vi "Serial Test Controller.vi"() -> ()   [LabVIEW 2012]
uses:
  Type/_RT Serial Command.ctl
  Type/_RT Command.ctl
  <vilib>/Utility/config.llb/Read Key (String).vi
  <vilib>/Utility/config.llb/NI_LVConfig.lvlib
panel:
  in  "Serial Property":T1[](array[typedef])=[{"Port Type"=0, "baud rate (9600)"=9600, "data bits (8)"=8, "stop bits (1)"=10, "parity (0:none)"=0, "DoRead"=TRUE, "Command"=""}, {"Port Type"=1, "baud rate (9600)"=9600, "data bits (8)"=8, "stop bits (1)"=10, "parity (0:none)"=0, "DoRead"=TRUE, "Command"=""}, {"Port Type"=2, "baud rate (9600)"=9600, "data bits (8)"=8, "stop bits (1)"=10, "parity (0:none)"=0, "DoRead"=TRUE, "Command"=""}] {"stop bits (1)" items=["1 bit"=10, "1.5 bits"=15, "2 bits"=20]; "parity (0:none)" items=["None", "Odd", "Even", "Mark", "Space"]; "data bits (8)" min=5 max=8 step=1; "Port Type" items=["RS485", "RS232-1", "RS232-2"]}
  in  "Tab":T2(tab)
  out "Reply":string
  in  "Command":string
  in  "Serial Port":u16(ring) items=["RS485", "RS232-1", "RS232-2"]
  in  "baud rate":u32=9600
  in  "parity":u16(ring) items=["None", "Odd", "Even", "Mark", "Space"]
  in  "stop bits":u16(ring)=10 items=["1 bit"=10, "1.5 bits"=15, "2 bits"=20]
  in  "data bits":u16=8 min=5 max=8 step=1
  in  "Send":bool
  in  "LC1 - Out1":bool
  in  "LC1 - Out2":bool
  in  "LC2 - Out1":bool
  in  "LC2 - Out2":bool
  out "LC1 - In":bool
  out "LC2 - In":bool
  in  "Update":bool
  in  "Read VAC":bool
  out "VAC Gauge Reading":i32
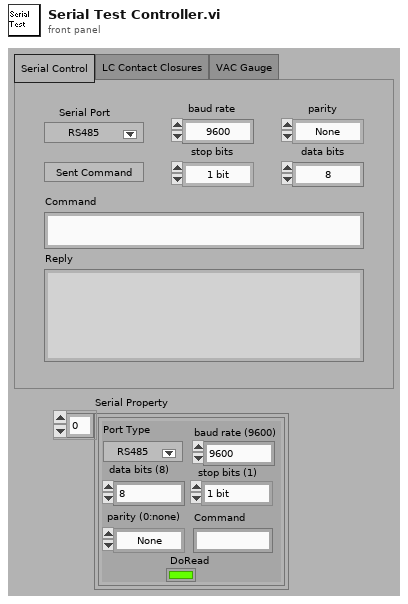
[diagram p1: front panel]
types:
  T1 = typedef "_RT Serial Command.ctl" = cluster{"Port Type":u16, "baud rate (9600)":u32, "data bits (8)":u16, "stop bits (1)":u16, "parity (0:none)":u16, "DoRead":bool, "Command":string}
  T2 = enum32{"Serial Control", "LC Contact Closures", "VAC Gauge"}
  T3 = typedef "_RT Command.ctl" = enum16{"Start", "Stop", "Runtime Update", "Get Data", "Get Info", "Get Status", "Get Param", "Get Config", "Get Table", "Read ADC", "Set Oscillator", "Update Config", "Update Table", "Set All Pol", "Set Pol and DC", "Set Max Mass", "Toggle RP", "Toggle EL", "Set PIC", "Initialize Turbo", "Send Turbo Comm", "Close Turbo", "P1", "P2", "P3", "Send Serial", "Set LC Out", "Get LC In", "Read VAC", "Test Table", "Toggle Power", "Get Startup", "Set Startup", "Get ADC Table", "Set ADC Table", "Get Brief Status", "Get Detail Status", "Auxiliary Update", "Set CC Logics", "Set CC Input Logics", "Ignore Error"}
  T4 = typedef "NI_LVConfig.lvlib/Config Data RefNum.ctl" = refnum<k1>
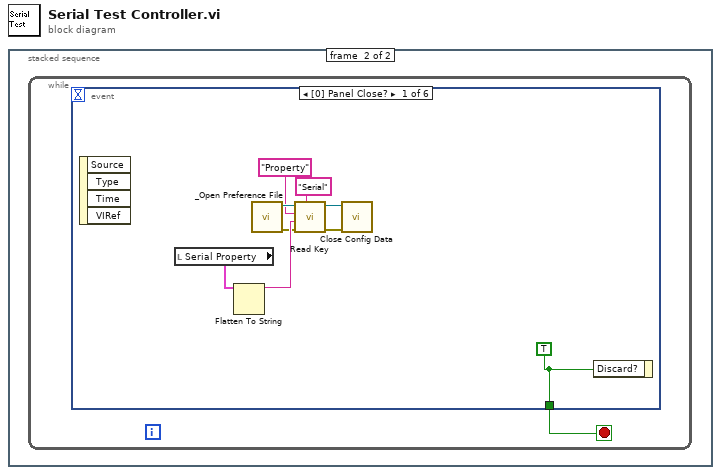
[diagram p0: block diagram]
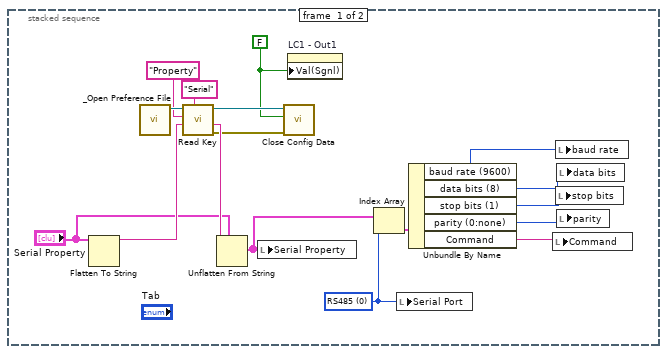
[diagram p2: hidden frame]
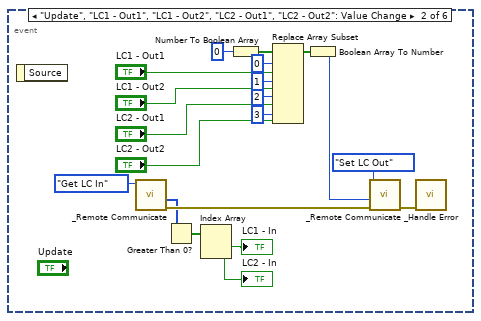
[diagram p3: hidden frame]
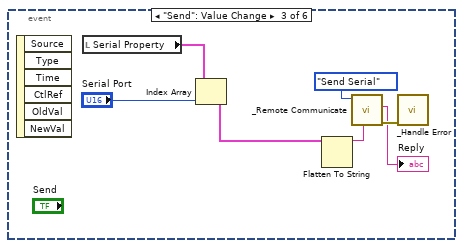
[diagram p4: hidden frame]
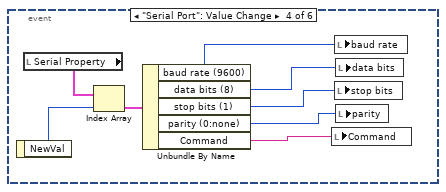
[diagram p5: hidden frame]
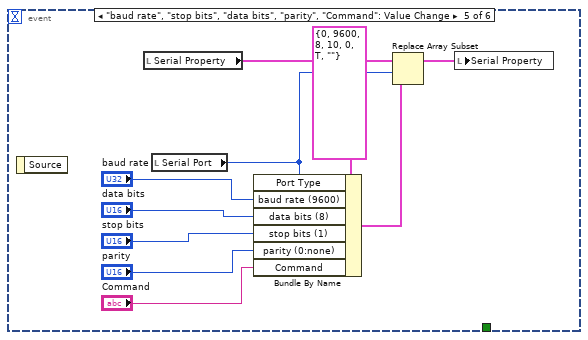
[diagram p6: hidden frame]
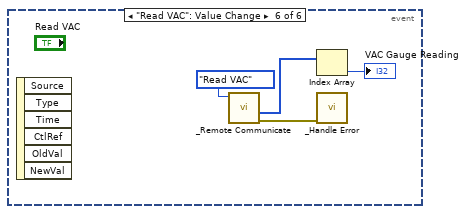
[diagram p7: hidden frame]
diagram:
  n1 = stacked-sequence {
    frame #0 {
      w7 = u16 0 items=["RS485", "RS232-1", "RS232-2"] ("Serial Port")
      w9 = FALSE ("write configuration file? (T)")
      n2 = Flatten To String(anything="Serial Property") -> (data string=w14:string)  [unwired: 1 in, 4 out]
      n3 = call "_Open Preference File.vi"() -> ("refnum"=w17:T4)  [unwired: 1 in, 6 out]
      n4 = call-poly <vilib>:"Read Key.vi"("section"="Serial", "default value"=w14, "key"="Property" ("section"), "refnum"=w17) -> ("error out"=w10:errorcluster, "value"=w13:string, "refnum out"=w11:T4)  [unwired: 2 in, 3 out]
      n5 = Unflatten From String(type="Serial Property", binary string=w13) -> (value=w8:T1[])  [unwired: 1 in, 4 out]
      n6 = local write "Serial Property"(w8) -> ()
      n7 = call <vilib>:"Close Config Data.vi"("error in (no error)"=w10, "write file if changed (T)"=w9, "refnum"=w11) -> ()  [unwired: 9 out]
      n8 = property on="LC1 - Out1" class="Bool (strict)"("Val(Sgnl)"=w9) -> ()  [unwired: 2 in, 2 out]
      n9 = Index Array(array=w8, index=w7) -> (element=w6:T1)
      n10 = local write "Serial Port"(w7) -> ()
      n11 = Unbundle By Name(w6) -> ("baud rate (9600)"=w5:u32, "data bits (8)"=w1:u16, "stop bits (1)"=w2:u16, "parity (0:none)"=w3:u16, "Command"=w4:string)
      n12 = local write "Command"(w4) -> ()
      n13 = local write "baud rate"(w5) -> ()
      n14 = local write "stop bits"(w2) -> ()
      n15 = local write "data bits"(w1) -> ()
      n16 = local write "parity"(w3) -> ()
    }
    frame #1 {
      n17 = while {
        stop <- w18 stop-if-true
        n18 = event shown="[0] Panel Close?" {
          selector: _ -> [_ _ _ _ _ _]
          dyn-events: _ -> [_ _ _ _ _ _]
          timeout: _ -> [_ _ _ _ _ _]
          tunnel: [w27 _ _ _ _ _] -> w18
          event Panel Close? {
            w27 = TRUE
            n19 = event-data() -> ()  [unwired: 5 out]
            n20 = local read "Serial Property"() -> (w21:T1[])
            n21 = Flatten To String(anything=w21) -> (data string=w20:string)  [unwired: 1 in, 4 out]
            n22 = call "_Open Preference File.vi"() -> ("error"=w19:errorcluster, "refnum"=w26:T4)  [unwired: 1 in, 5 out]
            n23 = call-poly <vilib>:"Read Key.vi"("section"="Serial", "error in (no error)"=w19, "default value"=w20, "key"="Property" ("section"), "refnum"=w26) -> ("error out"=w22:errorcluster, "refnum out"=w23:T4)  [unwired: 1 in, 4 out]
            n24 = call <vilib>:"Close Config Data.vi"("error in (no error)"=w22, "refnum"=w23) -> ()  [unwired: 1 in, 9 out]
            n25 = event-data("Discard?"=w27) -> ()  [unwired: 1 in, 1 out]
          }
          event "Update", "LC1 - Out1", "LC1 - Out2", "LC2 - Out1", "LC2 - Out2": Value Change {
            n26 = event-data() -> ()  [unwired: 2 out]
            n27 = call "_Remote Communicate.vi"("Command"=_RT_Command."Get LC In") -> ("error out"=w44:errorcluster, "Data Array"=w43:i32[])  [unwired: 5 in, 2 out]
            n28 = Greater Than 0?(x=w43) -> (x > 0?=w42:bool[])
            n29 = Index Array(array=w42) -> (element #1=→"LC1 - In":bool, element #2=→"LC2 - In":bool)  [unwired: 2 in]
            n30 = Number To Boolean Array(number=u16 0) -> (Boolean array=w38:bool[])
            n31 = Replace Array Subset(array=w38, new element #1="LC1 - Out1", index #1=0 ("index"), new element #2="LC1 - Out2", index #2=1 ("index"), new element #3="LC2 - Out1", index #3=2 ("index"), new element #4="LC2 - Out2", index #4=3 ("index")) -> (w35:bool[])
            n32 = Boolean Array To Number(Boolean array=w35) -> (number=w28:u16)
            n33 = call "_Remote Communicate.vi"("error in (no error)"=w44, "DC Param"=w28, "Command"=_RT_Command."Set LC Out") -> ("error out"=w46:errorcluster)  [unwired: 3 in, 3 out]
            n34 = call "_Handle Error.vi"("error in (no error)"=w46) -> ()  [unwired: 2 in, 5 out]
          }
          event "Send": Value Change {
            n35 = event-data() -> ()  [unwired: 7 out]
            n36 = local read "Serial Property"() -> (w50:T1[])
            n37 = Index Array(array=w50, index="Serial Port") -> (element=w48:T1)
            n38 = Flatten To String(anything=w48) -> (data string=w54:string)  [unwired: 1 in, 4 out]
            n39 = call "_Remote Communicate.vi"("String"=w54, "Command"=_RT_Command."Send Serial") -> ("error out"=w52:errorcluster, "Info"=→"Reply":string)  [unwired: 4 in, 2 out]
            n40 = call "_Handle Error.vi"("error in (no error)"=w52) -> ()  [unwired: 2 in, 5 out]
          }
          event "Serial Port": Value Change {
            n41 = event-data() -> ("NewVal"=w62:u16)  [unwired: 1 out]
            n42 = local read "Serial Property"() -> (w61:T1[])
            n43 = Index Array(array=w61, index=w62) -> (element=w60:T1)
            n44 = Unbundle By Name(w60) -> ("baud rate (9600)"=w59:u32, "data bits (8)"=w55:u16, "stop bits (1)"=w56:u16, "parity (0:none)"=w57:u16, "Command"=w58:string)
            n45 = local write "Command"(w58) -> ()
            n46 = local write "baud rate"(w59) -> ()
            n47 = local write "stop bits"(w56) -> ()
            n48 = local write "data bits"(w55) -> ()
            n49 = local write "parity"(w57) -> ()
          }
          event "baud rate", "stop bits", "data bits", "parity", "Command": Value Change {
            n50 = event-data() -> ()  [unwired: 2 out]
            n51 = local read "Serial Property"() -> (w72:T1[])
            n52 = local read "Serial Port"() -> (w70:u16)
            n53 = Bundle By Name(cluster=T1 {"Port Type"=0, "baud rate (9600)"=9600, "data bits (8)"=8, "stop bits (1)"=10, "parity (0:none)"=0, "DoRead"=TRUE, "Command"=""} ("Serial Command"), "Port Type"=w70, "baud rate (9600)"="baud rate", "data bits (8)"="data bits", "stop bits (1)"="stop bits", "parity (0:none)"="parity", "Command"="Command") -> (w68:T1)
            n54 = Replace Array Subset(array=w72, new element=w68, index=w70) -> (w71:T1[])
            n55 = local write "Serial Property"(w71) -> ()
          }
          event "Read VAC": Value Change {
            n56 = event-data() -> ()  [unwired: 7 out]
            n57 = call "_Remote Communicate.vi"("Command"=_RT_Command."Read VAC") -> ("error out"=w75:errorcluster, "Data Array"=w74:i32[])  [unwired: 5 in, 2 out]
            n58 = Index Array(array=w74) -> (element=→"VAC Gauge Reading":i32)  [unwired: 1 in]
            n59 = call "_Handle Error.vi"("error in (no error)"=w75) -> ()  [unwired: 2 in, 5 out]
          }
        }
      }
    }
  }
